vi "AnyBuilderBeginNestedMessage.vi"(8 "error in":errorcluster, 10 "protobufId":i32, 11 "gRPCid in":T1) -> (0 "error out":errorcluster, 2 "Nested ID":T1, 3 "gRPCid out":T1)   [LabVIEW 2019, in "grpc-lvsupport.lvlib"]
uses:
  grpc-lvsupport.lvlib
  Shared/grpcId.ctl
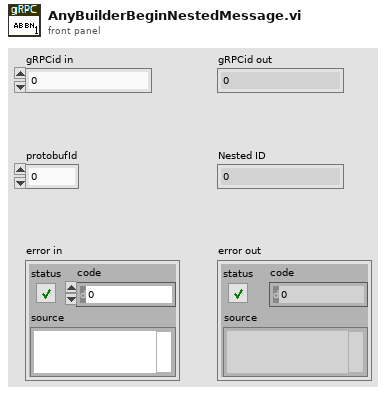
[diagram p1: front panel]
types:
  T1 = typedef "grpc-lvsupport.lvlib/grpcId.ctl" = u64
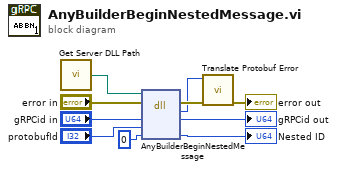
[diagram p0: block diagram]
diagram:
  n1 = call "Get Server DLL Path.vi"() -> ("Server dll path"=w5:path)
  n2 = dll-call lib="?" fn="AnyBuilderBeginNestedMessage"(path in=w5, error in="error in", "builderId"="gRPCid in", "protobufId"="protobufId", "nestedId"=u64 0) -> (error out=w9:errorcluster, "return type"=w1:i32, "builderId"=→"gRPCid out":u64, "nestedId"=→"Nested ID":u64)  [unwired: 2 in, 1 out]
  n3 = call "Translate Protobuf Error.vi"("error in"=w9, "Error Code"=w1) -> ("error out"=→"error out":errorcluster)  [unwired: 9 in]
